vi "(TestVI)DW7802 PWL Ramp Map Test 2.vi"() -> ()   [LabVIEW 2020]
uses:
  <vilib>/Utility/file.llb/Read Delimited Spreadsheet (string).vi
panel:
  out "추가된 배열":string[][](array[string])
  out "Scaling Ratio":dbl
  out "Delta_Amplitude":dbl
  in  "Cycle_N":u8=1 min=1 max=20
  in  "p(x+1)":dbl(ring) items=["0"=0.0, "10"=10.0, "20"=20.0, "30"=30.0, "40"=40.0, "50"=50.0, "60"=60.0, "70"=70.0, "80"=80.0, "90"=90.0, "100"=100.0]
  in  "p(x)":dbl(ring) items=["0"=0.0, "10"=10.0, "20"=20.0, "30"=30.0, "40"=40.0, "50"=50.0, "60"=60.0, "70"=70.0, "80"=80.0, "90"=90.0, "100"=100.0]
  out "all rows":string[][](array[string])=[["0", "0.000 ", "0.000 ", "00", "00", "", "0", "0", "0", "00", "00", "0", "0", "00", "00", "0", "0.000 ", "0.000 ", "", "", "", ""], ["1", "0.781 ", "0.260 ", "01", "00", "", "1", "1", "128", "7F", "7F", "127", "127", "7F", "7F", "0.1", "100.000 ", "100.000 ", "", "", "", ""], ["2", "1.563 ", "0.272 ", "02", "00", "", "2", "1", "128", "7F", "7F", "127", "127", "7F", "7F", "0.1", "100.000 ", "100.000 ", "", "", "", ""], ["3", "2.344 ", "0.285 ", "03", "00", "", "3", "1", "128", "7F", "7F", "127", "127", "7F", "7F", "0.1", "100.000 ", "100.000 ", "", "", "", ""], ["4", "3.125 ", "0.299 ", "04", "00", "", "4", "1", "128", "7F", "7F", "127", "127", "7F", "7F", "0.1", "100.000 ", "100.000 ", "", "", "", ""], ["5", "3.906 ", "0.313 ", "05", "00", "", "5", "1", "128", "7F", "7F", "127", "127", "7F", "7F", "0.1", "100.000 ", "100.000 ", "", "", "", ""], ["6", "4.688 ", "0.328 ", "06", "00", "", "6", "1", "128", "7F", "7F", "127", "127", "7F", "7F", "0.1", "100.000 ", "100.000 ", "", "", "", ""], ["7", "5.469 ", "0.344 ", "07", "00", "", "7", "1", "128", "7F", "7F", "127", "127", "7F", "7F", "0.1", "100.000 ", "100.000 ", "", "", "", ""], ["8", "6.250 ", "0.361 ", "08", "00", "", "8", "1", "128", "7F", "7F", "127", "127", "7F", "7F", "0.1", "100.000 ", "100.000 ", "", "", "", ""], ["9", "7.031 ", "0.378 ", "09", "00", "", "9", "1", "128", "7F", "7F", "127", "127", "7F", "7F", "0.1", "100.000 ", "100.000 ", "", "", "", ""], ["10", "7.813 ", "0.396 ", "0A", "01", "", "10", "1", "128", "7F", "7F", "127", "127", "7F", "7F", "0.1", "100.000 ", "100.000 ", "", "", "", ""], ["11", "8.594 ", "0.415 ", "0B", "01", "", "11", "1", "128", "7F", "7F", "127", "127", "7F", "7F", "0.1", "100.000 ", "100.000 ", "", "", "", ""], ["12", "9.375 ", "0.435 ", "0C", "01", "", "12", "1", "128", "7F", "7F", "127", "127", "7F", "7F", "0.1", "100.000 ", "100.000 ", "", "", "", ""], ["13", "10.156 ", "0.456 ", "0D", "01", "", "13", "1", "128", "7F", "7F", "127", "127", "7F", "7F", "0.2", "100.000 ", "100.000 ", "", "", "", ""], ["14", "10.938 ", "0.478 ", "0E", "01", "", "14", "1", "128", "7F", "7F", "127", "127", "7F", "7F", "0.2", "100.000 ", "100.000 ", "", "", "", ""], ["15", "11.719 ", "0.501 ", "0F", "01", "", "15", "1", "128", "7F", "7F", "127", "127", "7F", "7F", "0.2", "100.000 ", "100.000 ", "", "", "", ""], ["16", "12.500 ", "0.525 ", "10", "01", "", "16", "1", "128", "7F", "7F", "127", "127", "7F", "7F", "0.2", "100.000 ", "100.000 ", "", "", "", ""], ["17", "13.281 ", "0.550 ", "11", "01", "", "17", "1", "128", "7F", "7F", "127", "127", "7F", "7F", "0.2", "100.000 ", "100.000 ", "", "", "", ""], ["18", "14.063 ", "0.576 ", "12", "01", "", "18", "1", "128", "7F", "7F", "127", "127", "7F", "7F", "0.2", "100.000 ", "100.000 ", "", "", "", ""], ["19", "14.844 ", "0.604 ", "13", "01", "", "19", "1", "128", "7F", "7F", "127", "127", "7F", "7F", "0.2", "100.000 ", "100.000 ", "", "", "", ""], ["20", "15.625 ", "0.633 ", "14", "01", "", "20", "1", "128", "7F", "7F", "127", "127", "7F", "7F", "0.2", "100.000 ", "100.000 ", "", "", "", ""], ["21", "16.406 ", "0.663 ", "15", "01", "", "21", "1", "128", "7F", "7F", "127", "127", "7F", "7F", "0.2", "100.000 ", "100.000 ", "", "", "", ""], ["22", "17.188 ", "0.695 ", "16", "01", "", "22", "1", "128", "7F", "7F", "127", "127", "7F", "7F", "0.2", "100.000 ", "100.000 ", "", "", "", ""], ["23", "17.969 ", "0.729 ", "17", "01", "", "23", "1", "128", "7F", "7F", "127", "127", "7F", "7F", "0.2", "100.000 ", "100.000 ", "", "", "", ""], ["24", "18.750 ", "0.764 ", "18", "01", "", "24", "1", "128", "7F", "7F", "127", "127", "7F", "7F", "0.2", "100.000 ", "100.000 ", "", "", "", ""], ["25", "19.531 ", "0.800 ", "19", "01", "", "25", "1", "128", "7F", "7F", "127", "127", "7F", "7F", "0.2", "100.000 ", "100.000 ", "", "", "", ""], ["26", "20.313 ", "0.839 ", "1A", "01", "", "26", "1", "128", "7F", "7F", "127", "127", "7F", "7F", "0.3", "100.000 ", "100.000 ", "", "", "", ""], ["27", "21.094 ", "0.879 ", "1B", "01", "", "27", "1", "128", "7F", "7F", "127", "127", "7F", "7F", "0.3", "100.000 ", "100.000 ", "", "", "", ""], ["28", "21.875 ", "0.921 ", "1C", "01", "", "28", "1", "128", "7F", "7F", "127", "127", "7F", "7F", "0.3", "100.000 ", "100.000 ", "", "", "", ""], ["29", "22.656 ", "0.965 ", "1D", "01", "", "29", "1", "128", "7F", "7F", "127", "127", "7F", "7F", "0.3", "100.000 ", "100.000 ", "", "", "", ""], ["30", "23.438 ", "1.011 ", "1E", "01", "", "30", "1", "128", "7F", "7F", "127", "127", "7F", "7F", "0.3", "100.000 ", "100.000 ", "", "", "", ""], ["31", "24.219 ", "1.060 ", "1F", "01", "", "31", "1", "128", "7F", "7F", "127", "127", "7F", "7F", "0.3", "100.000 ", "100.000 ", "", "", "", ""], ["32", "25.000 ", "1.111 ", "20", "01", "", "32", "1", "128", "7F", "7F", "127", "127", "7F", "7F", "0.3", "100.000 ", "100.000 ", "", "", "", ""], ["33", "25.781 ", "1.164 ", "21", "01", "", "33", "1", "128", "7F", "7F", "127", "127", "7F", "7F", "0.3", "100.000 ", "100.000 ", "", "", "", ""], ["34", "26.563 ", "1.220 ", "22", "02", "", "34", "1", "128", "7F", "7F", "127", "127", "7F", "7F", "0.3", "100.000 ", "100.000 ", "", "", "", ""], ["35", "27.344 ", "1.279 ", "23", "02", "", "35", "1", "128", "7F", "7F", "127", "127", "7F", "7F", "0.3", "100.000 ", "100.000 ", "", "", "", ""], ["36", "28.125 ", "1.340 ", "24", "02", "", "36", "1", "128", "7F", "7F", "127", "127", "7F", "7F", "0.3", "100.000 ", "100.000 ", "", "", "", ""], ["37", "28.906 ", "1.404 ", "25", "02", "", "37", "1", "128", "7F", "7F", "127", "127", "7F", "7F", "0.3", "100.000 ", "100.000 ", "", "", "", ""], ["38", "29.688 ", "1.472 ", "26", "02", "", "38", "1", "128", "7F", "7F", "127", "127", "7F", "7F", "0.3", "100.000 ", "100.000 ", "", "", "", ""], ["39", "30.469 ", "1.542 ", "27", "02", "", "39", "1", "128", "7F", "7F", "127", "127", "7F", "7F", "0.4", "100.000 ", "100.000 ", "", "", "", ""], ["40", "31.250 ", "1.616 ", "28", "02", "", "40", "1", "128", "7F", "7F", "127", "127", "7F", "7F", "0.4", "100.000 ", "100.000 ", "", "", "", ""], ["41", "32.031 ", "1.694 ", "29", "02", "", "41", "1", "128", "7F", "7F", "127", "127", "7F", "7F", "0.4", "100.000 ", "100.000 ", "", "", "", ""], ["42", "32.813 ", "1.775 ", "2A", "02", "", "42", "1", "128", "7F", "7F", "127", "127", "7F", "7F", "0.4", "100.000 ", "100.000 ", "", "", "", ""], ["43", "33.594 ", "1.860 ", "2B", "02", "", "43", "1", "128", "7F", "7F", "127", "127", "7F", "7F", "0.4", "100.000 ", "100.000 ", "", "", "", ""], ["44", "34.375 ", "1.950 ", "2C", "02", "", "44", "1", "128", "7F", "7F", "127", "127", "7F", "7F", "0.4", "100.000 ", "100.000 ", "", "", "", ""], ["45", "35.156 ", "2.043 ", "2D", "03", "", "45", "1", "128", "7F", "7F", "127", "127", "7F", "7F", "0.4", "100.000 ", "100.000 ", "", "", "", ""], ["46", "35.938 ", "2.141 ", "2E", "03", "", "46", "1", "128", "7F", "7F", "127", "127", "7F", "7F", "0.4", "100.000 ", "100.000 ", "", "", "", ""], ["47", "36.719 ", "2.244 ", "2F", "03", "", "47", "1", "128", "7F", "7F", "127", "127", "7F", "7F", "0.4", "100.000 ", "100.000 ", "", "", "", ""], ["48", "37.500 ", "2.352 ", "30", "03", "", "48", "1", "128", "7F", "7F", "127", "127", "7F", "7F", "0.4", "100.000 ", "100.000 ", "", "", "", ""], ["49", "38.281 ", "2.465 ", "31", "03", "", "49", "1", "128", "7F", "7F", "127", "127", "7F", "7F", "0.4", "100.000 ", "100.000 ", "", "", "", ""], ["50", "39.063 ", "2.583 ", "32", "03", "", "50", "1", "128", "7F", "7F", "127", "127", "7F", "7F", "0.4", "100.000 ", "100.000 ", "", "", "", ""], ["51", "39.844 ", "2.707 ", "33", "03", "", "51", "1", "128", "7F", "7F", "127", "127", "7F", "7F", "0.4", "100.000 ", "100.000 ", "", "", "", ""], ["52", "40.625 ", "2.837 ", "34", "04", "", "52", "1", "128", "7F", "7F", "127", "127", "7F", "7F", "0.5", "100.000 ", "100.000 ", "", "", "", ""], ["53", "41.406 ", "2.973 ", "35", "04", "", "53", "1", "128", "7F", "7F", "127", "127", "7F", "7F", "0.5", "100.000 ", "100.000 ", "", "", "", ""], ["54", "42.188 ", "3.116 ", "36", "04", "", "54", "1", "128", "7F", "7F", "127", "127", "7F", "7F", "0.5", "100.000 ", "100.000 ", "", "", "", ""], ["55", "42.969 ", "3.265 ", "37", "04", "", "55", "1", "128", "7F", "7F", "127", "127", "7F", "7F", "0.5", "100.000 ", "100.000 ", "", "", "", ""], ["56", "43.750 ", "3.422 ", "38", "04", "", "56", "1", "128", "7F", "7F", "127", "127", "7F", "7F", "0.5", "100.000 ", "100.000 ", "", "", "", ""], ["57", "44.531 ", "3.586 ", "39", "05", "", "57", "1", "128", "7F", "7F", "127", "127", "7F", "7F", "0.5", "100.000 ", "100.000 ", "", "", "", ""], ["58", "45.313 ", "3.758 ", "3A", "05", "", "58", "1", "128", "7F", "7F", "127", "127", "7F", "7F", "0.5", "100.000 ", "100.000 ", "", "", "", ""], ["59", "46.094 ", "3.938 ", "3B", "05", "", "59", "1", "128", "7F", "7F", "127", "127", "7F", "7F", "0.5", "100.000 ", "100.000 ", "", "", "", ""], ["60", "46.875 ", "4.127 ", "3C", "05", "", "60", "1", "128", "7F", "7F", "127", "127", "7F", "7F", "0.5", "100.000 ", "100.000 ", "", "", "", ""], ["61", "47.656 ", "4.326 ", "3D", "05", "", "61", "1", "128", "7F", "7F", "127", "127", "7F", "7F", "0.5", "100.000 ", "100.000 ", "", "", "", ""], ["62", "48.438 ", "4.533 ", "3E", "06", "", "62", "1", "128", "7F", "7F", "127", "127", "7F", "7F", "0.5", "100.000 ", "100.000 ", "", "", "", ""], ["63", "49.219 ", "4.751 ", "3F", "06", "", "63", "1", "128", "7F", "7F", "127", "127", "7F", "7F", "0.5", "100.000 ", "100.000 ", "", "", "", ""], ["64", "50.000 ", "4.979 ", "40", "06", "", "64", "1", "128", "7F", "7F", "127", "127", "7F", "7F", "0.5", "100.000 ", "100.000 ", "", "", "", ""], ["65", "50.781 ", "5.218 ", "40", "07", "", "65", "1", "128", "7F", "7F", "127", "127", "7F", "7F", "0.6", "100.000 ", "100.000 ", "", "", "", ""], ["66", "51.563 ", "5.468 ", "41", "07", "", "66", "1", "128", "7F", "7F", "127", "127", "7F", "7F", "0.6", "100.000 ", "100.000 ", "", "", "", ""], ["67", "52.344 ", "5.730 ", "42", "07", "", "67", "1", "128", "7F", "7F", "127", "127", "7F", "7F", "0.6", "100.000 ", "100.000 ", "", "", "", ""], ["68", "53.125 ", "6.005 ", "43", "08", "", "68", "1", "128", "7F", "7F", "127", "127", "7F", "7F", "0.6", "100.000 ", "100.000 ", "", "", "", ""], ["69", "53.906 ", "6.294 ", "44", "08", "", "69", "1", "128", "7F", "7F", "127", "127", "7F", "7F", "0.6", "100.000 ", "100.000 ", "", "", "", ""], ["70", "54.688 ", "6.596 ", "45", "08", "", "70", "1", "128", "7F", "7F", "127", "127", "7F", "7F", "0.6", "100.000 ", "100.000 ", "", "", "", ""], ["71", "55.469 ", "6.912 ", "46", "09", "", "71", "1", "128", "7F", "7F", "127", "127", "7F", "7F", "0.6", "100.000 ", "100.000 ", "", "", "", ""], ["72", "56.250 ", "7.244 ", "47", "09", "", "72", "1", "128", "7F", "7F", "127", "127", "7F", "7F", "0.6", "100.000 ", "100.000 ", "", "", "", ""], ["73", "57.031 ", "7.592 ", "48", "0A", "", "73", "1", "128", "7F", "7F", "127", "127", "7F", "7F", "0.6", "100.000 ", "100.000 ", "", "", "", ""], ["74", "57.813 ", "7.956 ", "49", "0A", "", "74", "1", "128", "7F", "7F", "127", "127", "7F", "7F", "0.6", "100.000 ", "100.000 ", "", "", "", ""], ["75", "58.594 ", "8.338 ", "4A", "0B", "", "75", "1", "128", "7F", "7F", "127", "127", "7F", "7F", "0.6", "100.000 ", "100.000 ", "", "", "", ""], ["76", "59.375 ", "8.738 ", "4B", "0B", "", "76", "1", "128", "7F", "7F", "127", "127", "7F", "7F", "0.6", "100.000 ", "100.000 ", "", "", "", ""], ["77", "60.156 ", "9.157 ", "4C", "0C", "", "77", "1", "128", "7F", "7F", "127", "127", "7F", "7F", "0.7", "100.000 ", "100.000 ", "", "", "", ""], ["78", "60.938 ", "9.597 ", "4D", "0C", "", "78", "1", "128", "7F", "7F", "127", "127", "7F", "7F", "0.7", "100.000 ", "100.000 ", "", "", "", ""], ["79", "61.719 ", "10.057 ", "4E", "0D", "", "79", "1", "128", "7F", "7F", "127", "127", "7F", "7F", "0.7", "100.000 ", "100.000 ", "", "", "", ""], ["80", "62.500 ", "10.540 ", "4F", "0D", "", "80", "1", "128", "7F", "7F", "127", "127", "7F", "7F", "0.7", "100.000 ", "100.000 ", "", "", "", ""], ["81", "63.281 ", "11.046 ", "50", "0E", "", "81", "1", "128", "7F", "7F", "127", "127", "7F", "7F", "0.7", "100.000 ", "100.000 ", "", "", "", ""], ["82", "64.063 ", "11.576 ", "51", "0F", "", "82", "1", "128", "7F", "7F", "127", "127", "7F", "7F", "0.7", "100.000 ", "100.000 ", "", "", "", ""], ["83", "64.844 ", "12.131 ", "52", "0F", "", "83", "1", "128", "7F", "7F", "127", "127", "7F", "7F", "0.7", "100.000 ", "100.000 ", "", "", "", ""], ["84", "65.625 ", "12.714 ", "53", "10", "", "84", "1", "128", "7F", "7F", "127", "127", "7F", "7F", "0.7", "100.000 ", "100.000 ", "", "", "", ""], ["85", "66.406 ", "13.324 ", "54", "11", "", "85", "1", "128", "7F", "7F", "127", "127", "7F", "7F", "0.7", "100.000 ", "100.000 ", "", "", "", ""], ["86", "67.188 ", "13.963 ", "55", "12", "", "86", "1", "128", "7F", "7F", "127", "127", "7F", "7F", "0.7", "100.000 ", "100.000 ", "", "", "", ""], ["87", "67.969 ", "14.633 ", "56", "13", "", "87", "1", "128", "7F", "7F", "127", "127", "7F", "7F", "0.7", "100.000 ", "100.000 ", "", "", "", ""], ["88", "68.750 ", "15.335 ", "57", "13", "", "88", "1", "128", "7F", "7F", "127", "127", "7F", "7F", "0.7", "100.000 ", "100.000 ", "", "", "", ""], ["89", "69.531 ", "16.071 ", "58", "14", "", "89", "1", "128", "7F", "7F", "127", "127", "7F", "7F", "0.7", "100.000 ", "100.000 ", "", "", "", ""], ["90", "70.313 ", "16.843 ", "59", "15", "", "90", "1", "128", "7F", "7F", "127", "127", "7F", "7F", "0.8", "100.000 ", "100.000 ", "", "", "", ""], ["91", "71.094 ", "17.651 ", "5A", "16", "", "91", "1", "128", "7F", "7F", "127", "127", "7F", "7F", "0.8", "100.000 ", "100.000 ", "", "", "", ""], ["92", "71.875 ", "18.498 ", "5B", "17", "", "92", "1", "128", "7F", "7F", "127", "127", "7F", "7F", "0.8", "100.000 ", "100.000 ", "", "", "", ""], ["93", "72.656 ", "19.386 ", "5C", "19", "", "93", "1", "128", "7F", "7F", "127", "127", "7F", "7F", "0.8", "100.000 ", "100.000 ", "", "", "", ""], ["94", "73.438 ", "20.316 ", "5D", "1A", "", "94", "1", "128", "7F", "7F", "127", "127", "7F", "7F", "0.8", "100.000 ", "100.000 ", "", "", "", ""], ["95", "74.219 ", "21.291 ", "5E", "1B", "", "95", "1", "128", "7F", "7F", "127", "127", "7F", "7F", "0.8", "100.000 ", "100.000 ", "", "", "", ""], ["96", "75.000 ", "22.313 ", "5F", "1C", "", "96", "1", "128", "7F", "7F", "127", "127", "7F", "7F", "0.8", "100.000 ", "100.000 ", "", "", "", ""], ["97", "75.781 ", "23.384 ", "60", "1E", "", "97", "1", "128", "7F", "7F", "127", "127", "7F", "7F", "0.8", "100.000 ", "100.000 ", "", "", "", ""], ["98", "76.563 ", "24.506 ", "61", "1F", "", "98", "1", "128", "7F", "7F", "127", "127", "7F", "7F", "0.8", "100.000 ", "100.000 ", "", "", "", ""], ["99", "77.344 ", "25.682 ", "62", "21", "", "99", "1", "128", "7F", "7F", "127", "127", "7F", "7F", "0.8", "100.000 ", "100.000 ", "", "", "", ""], ["100", "78.125 ", "26.915 ", "63", "22", "", "100", "1", "128", "7F", "7F", "127", "127", "7F", "7F", "0.8", "100.000 ", "100.000 ", "", "", "", ""], ["101", "78.906 ", "28.206 ", "64", "24", "", "101", "1", "128", "7F", "7F", "127", "127", "7F", "7F", "0.8", "100.000 ", "100.000 ", "", "", "", ""], ["102", "79.688 ", "29.560 ", "65", "26", "", "102", "1", "128", "7F", "7F", "127", "127", "7F", "7F", "0.8", "100.000 ", "100.000 ", "", "", "", ""], ["103", "80.469 ", "30.979 ", "66", "27", "", "103", "1", "128", "7F", "7F", "127", "127", "7F", "7F", "0.9", "100.000 ", "100.000 ", "", "", "", ""], ["104", "81.250 ", "32.465 ", "67", "29", "", "104", "1", "128", "7F", "7F", "127", "127", "7F", "7F", "0.9", "100.000 ", "100.000 ", "", "", "", ""], ["105", "82.031 ", "34.023 ", "68", "2B", "", "105", "1", "128", "7F", "7F", "127", "127", "7F", "7F", "0.9", "100.000 ", "100.000 ", "", "", "", ""], ["106", "82.813 ", "35.656 ", "69", "2D", "", "106", "1", "128", "7F", "7F", "127", "127", "7F", "7F", "0.9", "100.000 ", "100.000 ", "", "", "", ""], ["107", "83.594 ", "37.367 ", "6A", "2F", "", "107", "1", "128", "7F", "7F", "127", "127", "7F", "7F", "0.9", "100.000 ", "100.000 ", "", "", "", ""], ["108", "84.375 ", "39.161 ", "6B", "32", "", "108", "1", "128", "7F", "7F", "127", "127", "7F", "7F", "0.9", "100.000 ", "100.000 ", "", "", "", ""], ["109", "85.156 ", "41.040 ", "6C", "34", "", "109", "1", "128", "7F", "7F", "127", "127", "7F", "7F", "0.9", "100.000 ", "100.000 ", "", "", "", ""], ["110", "85.938 ", "43.009 ", "6D", "37", "", "110", "1", "128", "7F", "7F", "127", "127", "7F", "7F", "0.9", "100.000 ", "100.000 ", "", "", "", ""], ["111", "86.719 ", "45.074 ", "6E", "39", "", "111", "1", "128", "7F", "7F", "127", "127", "7F", "7F", "0.9", "100.000 ", "100.000 ", "", "", "", ""], ["112", "87.500 ", "47.237 ", "6F", "3C", "", "112", "1", "128", "7F", "7F", "127", "127", "7F", "7F", "0.9", "100.000 ", "100.000 ", "", "", "", ""], ["113", "88.281 ", "49.504 ", "70", "3F", "", "113", "1", "128", "7F", "7F", "127", "127", "7F", "7F", "0.9", "100.000 ", "100.000 ", "", "", "", ""], ["114", "89.063 ", "51.879 ", "71", "42", "", "114", "1", "128", "7F", "7F", "127", "127", "7F", "7F", "0.9", "100.000 ", "100.000 ", "", "", "", ""], ["115", "89.844 ", "54.369 ", "72", "45", "", "115", "1", "128", "7F", "7F", "127", "127", "7F", "7F", "0.9", "100.000 ", "100.000 ", "", "", "", ""], ["116", "90.625 ", "56.978 ", "73", "48", "", "116", "1", "128", "7F", "7F", "127", "127", "7F", "7F", "1", "100.000 ", "100.000 ", "", "", "", ""], ["117", "91.406 ", "59.713 ", "74", "4C", "", "117", "1", "128", "7F", "7F", "127", "127", "7F", "7F", "1", "100.000 ", "100.000 ", "", "", "", ""], ["118", "92.188 ", "62.578 ", "75", "4F", "", "118", "1", "128", "7F", "7F", "127", "127", "7F", "7F", "1", "100.000 ", "100.000 ", "", "", "", ""], ["119", "92.969 ", "65.582 ", "76", "53", "", "119", "1", "128", "7F", "7F", "127", "127", "7F", "7F", "1", "100.000 ", "100.000 ", "", "", "", ""], ["120", "93.750 ", "68.729 ", "77", "57", "", "120", "1", "128", "7F", "7F", "127", "127", "7F", "7F", "1", "100.000 ", "100.000 ", "", "", "", ""], ["121", "94.531 ", "72.027 ", "78", "5B", "", "121", "1", "128", "7F", "7F", "127", "127", "7F", "7F", "1", "100.000 ", "100.000 ", "", "", "", ""], ["122", "95.313 ", "75.484 ", "79", "60", "", "122", "1", "128", "7F", "7F", "127", "127", "7F", "7F", "1", "100.000 ", "100.000 ", "", "", "", ""], ["123", "96.094 ", "79.107 ", "7A", "64", "", "123", "1", "128", "7F", "7F", "127", "127", "7F", "7F", "1", "100.000 ", "100.000 ", "", "", "", ""], ["124", "96.875 ", "82.903 ", "7B", "69", "", "124", "1", "128", "7F", "7F", "127", "127", "7F", "7F", "1", "100.000 ", "100.000 ", "", "", "", ""], ["125", "97.656 ", "86.882 ", "7C", "6E", "", "125", "1", "128", "7F", "7F", "127", "127", "7F", "7F", "1", "100.000 ", "100.000 ", "", "", "", ""], ["126", "98.438 ", "91.051 ", "7D", "74", "", "126", "1", "128", "7F", "7F", "127", "127", "7F", "7F", "1", "100.000 ", "100.000 ", "", "", "", ""], ["127", "99.219 ", "95.421 ", "7E", "79", "", "127", "1", "128", "7F", "7F", "127", "127", "7F", "7F", "1", "100.000 ", "100.000 ", "", "", "", ""], ["128", "100.000 ", "100.000 ", "7F", "7F", "", "128", "1", "128", "7F", "7F", "127", "127", "7F", "7F", "1", "100.000 ", "100.000 ", "", "", "", ""]] caption="모든 행"
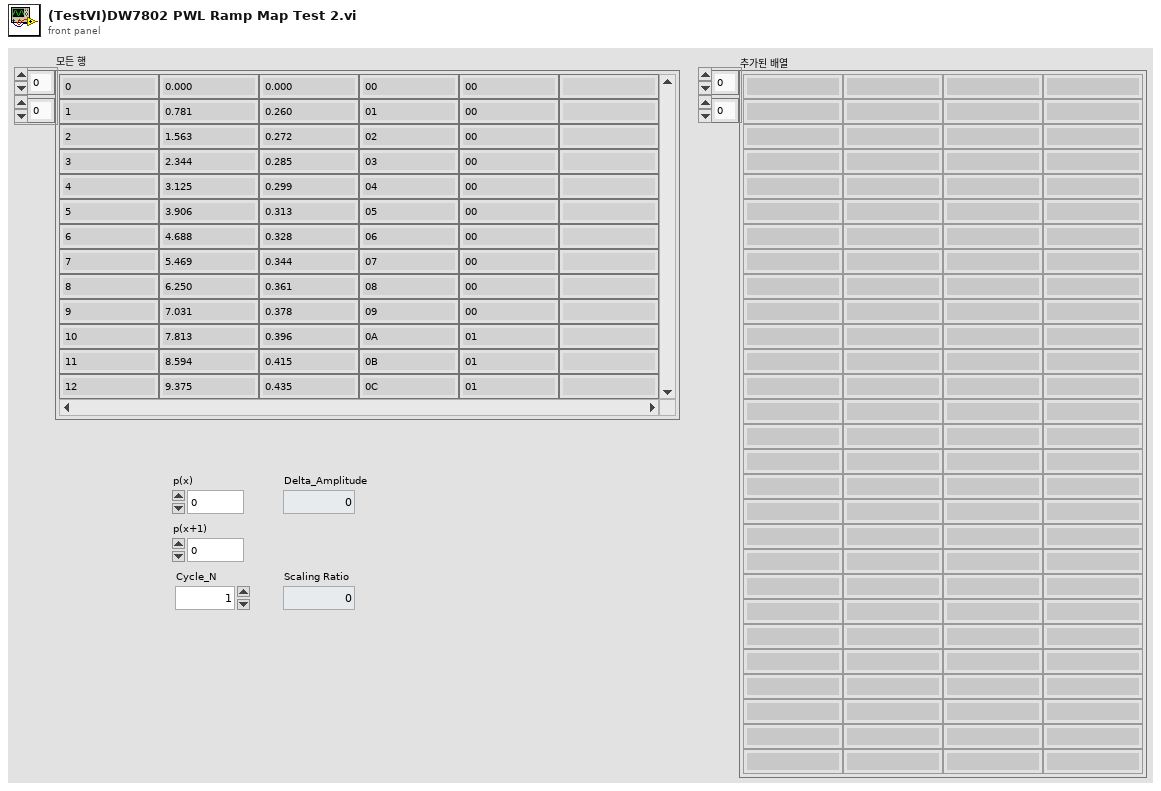
[diagram p1: front panel]
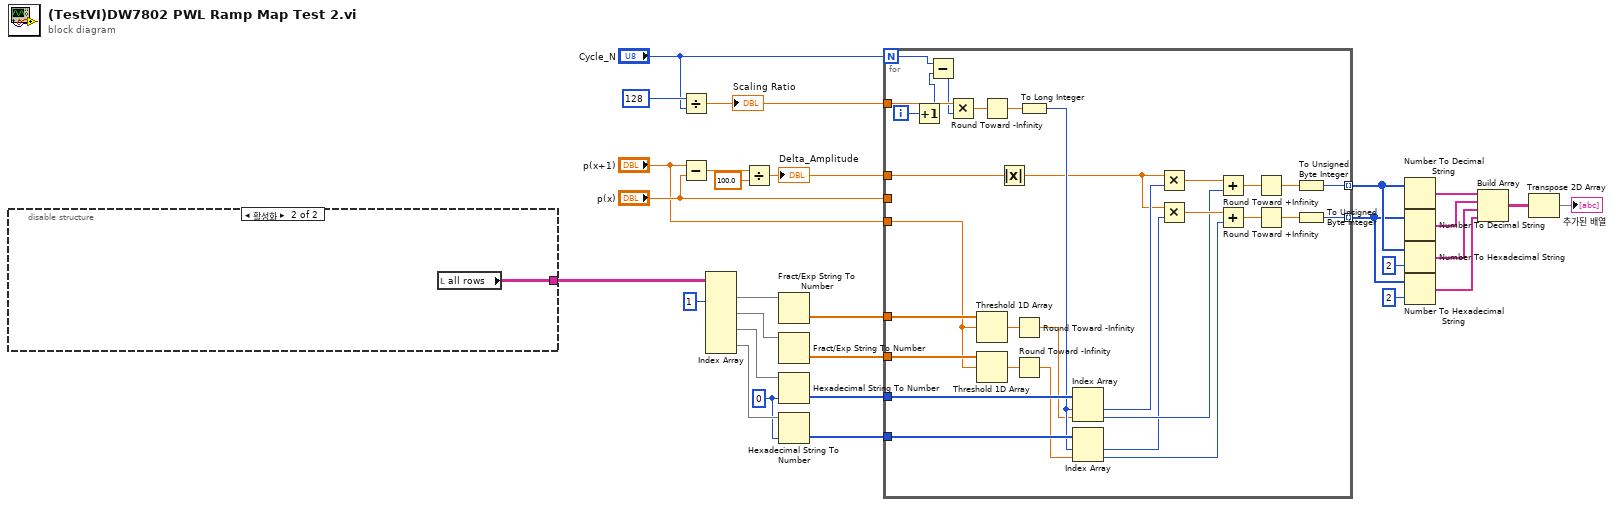
[diagram p0: block diagram]
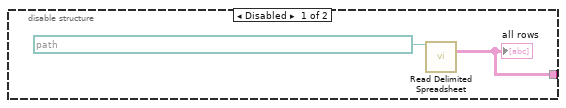
[diagram p2: hidden frame]
diagram:
  w26 = u8 0
  n1 = disable-structure shown="활성화" {
    disable-tunnel: [w30 w32] -> w29
    frame Disabled {
      n2 = call-poly <vilib>:"Read Delimited Spreadsheet.vi"("file path (dialog if empty)"=path "C:/Users/ParkHongSun/Desktop/복사본 DW7802_V5_220526.txt") -> ("all rows"=w30:string[][])  [unwired: 9 in, 5 out]
      "all rows" <- w30
    }
    frame Enabled {
      n3 = local read "all rows"() -> (w32:string[][])
    }
  }
  n4 = Divide(x=u8 128 ("y"), y="Cycle_N") -> (x/y=w23:dbl)
  "Scaling Ratio" <- w23
  n5 = Subtract(x="p(x+1)", y="p(x)") -> (x-y=w20:dbl)
  n6 = Index Array(array=w29, index (col) #1=1 ("비활성화된 인덱스 (열)")) -> (element #1=w19:string[], element #2=w18:string[], element #3=w28:string[], element #4=w27:string[])  [unwired: 7 in]
  n7 = Divide(x=w20, y=100.0) -> (x/y=w15:dbl)
  "Delta_Amplitude" <- w15
  n8 = Fract/Exp String To Number(string=w19) -> (number=w17:dbl[])  [unwired: 3 in, 1 out]
  n9 = Fract/Exp String To Number(string=w18) -> (number=w16:dbl[])  [unwired: 3 in, 1 out]
  n10 = Hexadecimal String To Number(string=w28, default (0uL)=w26) -> (number=w22:u8[])  [unwired: 1 in, 1 out]
  n11 = Hexadecimal String To Number(string=w27, default (0uL)=w26) -> (number=w21:u8[])  [unwired: 1 in, 1 out]
  n12 = for {
    N: "Cycle_N" -> [w39]
    tunnel: w23 -> [w63]
    tunnel: w22 -> [w62]
    tunnel: w21 -> [w61]
    tunnel: w15 -> [w37]
    tunnel: w17 -> [w56]
    tunnel: w16 -> [w55]
    tunnel: [w46] -> w13 mode=indexing
    tunnel: [w45] -> w12 mode=indexing
    tunnel: "p(x)" -> [_]
    tunnel: "p(x+1)" -> [w34]
    i -> [w38]
    n13 = Increment(x=w38) -> (x+1=w33:i32)
    n14 = Subtract(x=w39, y=w33) -> (x-y=w36:i32)
    n15 = Multiply(x=w63, y=w36) -> (x*y=w60:dbl)
    n16 = Threshold 1D Array(2:w34, 3:w56) -> (0:w53:dbl)  [unwired: 1 in]
    n17 = Threshold 1D Array(2:w34, 3:w55) -> (0:w54:dbl)  [unwired: 1 in]
    n18 = Round Toward -Infinity(1:w60) -> (0:w59:dbl)
    n19 = Absolute Value(x=w37) -> (abs(x)=w35:dbl)
    n20 = Round Toward -Infinity(1:w53) -> (0:w52:dbl)
    n21 = Round Toward -Infinity(1:w54) -> (0:w51:dbl)
    n22 = To Long Integer(number=w59) -> (32bit integer=w58:i32)
    n23 = Index Array(array=w62, index #1=w58, index #2=w52) -> (element #1=w57:u8, element #2=w48:u8)
    n24 = Index Array(array=w61, index #1=w58, index #2=w51) -> (element #1=w47:u8, element #2=w44:u8)
    n25 = Multiply(x=w35, y=w57) -> (x*y=w50:dbl)
    n26 = Multiply(x=w35, y=w47) -> (x*y=w49:dbl)
    n27 = Add(x=w50, y=w48) -> (x+y=w43:dbl)
    n28 = Add(x=w49, y=w44) -> (x+y=w42:dbl)
    n29 = Round Toward +Infinity(x=w43) -> (ceil(x): smallest int >= x=w41:dbl)
    n30 = Round Toward +Infinity(x=w42) -> (ceil(x): smallest int >= x=w40:dbl)
    n31 = To Unsigned Byte Integer(number=w41) -> (unsigned 8bit integer=w46:u8)
    n32 = To Unsigned Byte Integer(number=w40) -> (unsigned 8bit integer=w45:u8)
  }
  n33 = Number To Decimal String(number=w13) -> (decimal integer string=w11:string[])  [unwired: 1 in]
  n34 = Number To Decimal String(number=w12) -> (decimal integer string=w10:string[])  [unwired: 1 in]
  n35 = Number To Hexadecimal String(1:i16 2 ("폭(-)"), 2:w13) -> (0:w9:string[])
  n36 = Number To Hexadecimal String(1:i16 2 ("폭(-)"), 2:w12) -> (0:w8:string[])
  n37 = Build Array(w11, w10, w9, w8) -> (w7:string[][])
  n38 = Transpose 2D Array(2D array=w7) -> (transposed array=→"추가된 배열":string[][])
